vi "ManageResultsOutOfRangeLabels.vi"(11 "Input Array 2":string[](array[string])) -> (3 "Input Array 3":string[](array[string]))   [LabVIEW 2013]
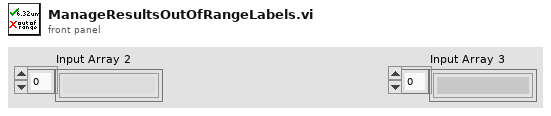
[diagram p1: front panel]
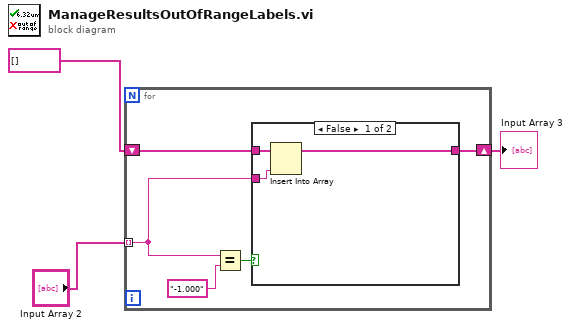
[diagram p0: block diagram]
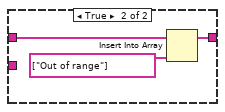
[diagram p2: hidden frame]
diagram:
  n1 = for {
    shift-right: [w7] -> w1
    shift-left: string[] [] ("Input Array 2") -> [w8]
    tunnel: "Input Array 2" -> [w4] mode=indexing
    n2 = Equal?(x=w4, y="-1.000") -> (x = y?=w5:bool)
    n3 = case shown="False" w5 {
      tunnel: w8 -> [w11 w14]
      tunnel: [w10 w13] -> w7
      tunnel: w4 -> [w9 _]
      frame False {
        n4 = Insert Into Array(array=w11, new element=w9) -> (w10:string[])  [unwired: 1 in]
      }
      frame True {
        n5 = Insert Into Array(array=w14, new element=string[] ["Out of range"] ("new element/subarray")) -> (w13:string[])  [unwired: 1 in]
      }
    }
  }
  "Input Array 3" <- w1
